vi "PH_PILS.set HV Warnlamp.vi"(0 "i ref in":refnum<vi>, 5 "error in (no error)":errorcluster) -> (14 "i ref out":refnum<vi>, 19 "error out":errorcluster)   [LabVIEW 2014, in "PH_PILS.lvlib"]
doc: "This VI switches flash lamp above door of the the HV-room in case of that the evacuation acqunoledgement is switched."
uses:
  PH_PILS.lvlib
  PH_Devices/PH_Beckhoff_PPMA-Rods/PH_Beckhoff_PPMA-Rods.lvlib
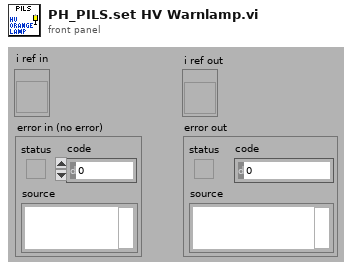
[diagram p1: front panel]
types:
  T1 = typedef "PH_PILS.lvlib/PH_PILS.i attribute.ctl" = cluster{"Boolean":cluster{"GUI Ref":refnum<vi>, "Status":i32}[], "GUI Refs Exp. Shutters":cluster{"1":refnum<vi>, "2":refnum<vi>, "3":refnum<vi>, "4":refnum<vi>}, "Tristate2Run GUI Refs":refnum<vi>[], "EO-Likes":cluster{"GUI Ref":refnum<vi>, "Status":i32}[], "Operation Mode":cluster{"Operation Mode":T2, "GUI":cluster{"Ref State":refnum<vi>, "Ref":refnum<vi>}, "Servicemode":cluster{"Tagname":string, "Status":i32}, "Labormode":cluster{"Tagname":string, "Status":i32}, "Searchmode":cluster{"Tagname":string, "Status":i32}, "Shotmode":cluster{"Tagname":string, "Status":i32}}, "Submode":cluster{"Submode":T3, "GUI":cluster{"Ref State":refnum<vi>, "Ref":refnum<vi>}, "Submode":cluster{"Tagname":string, "Status":i32}}, "Experiment":cluster{"Experiment":enum16{"unknown", "intern", "4 (Z6)", "3", "2", "1"}, "GUI":cluster{"Ref State":refnum<vi>, "Ref":refnum<vi>}, "intern":cluster{"Tagname":string, "Status":i32}, "Exp 4":cluster{"Tagname":string, "Status":i32}, "Exp 3":cluster{"Tagname":string, "Status":i32}, "Exp 2":cluster{"Tagname":string, "Status":i32}, "Exp 1":cluster{"Tagname":string, "Status":i32}}, "TristateNormal":cluster{"GUI Ref":refnum<vi>, "Status":i32}[], "Door Tags":cluster{"GUI Ref":refnum<vi>, "Status":i32}[], "GUIlessTags":cluster{"Name":string, "Status":i32}[], "Beamline GUI Refs":refnum<vi>[], "Special Boolean":cluster{"GUI Ref":refnum<vi>, "Status":i32}[], "Laserpower":cluster{"GUI Ref":refnum<vi>, "Status":i32}[], "Shutter":cluster{"GUI Ref":refnum<vi>, "Status":i32}[], "Tristate EO Like":cluster{"GUI Ref":refnum<vi>, "Status":i32}[], "PP":cluster{"GUI Ref":refnum<vi>, "Status":i32, "Head Ref":refnum<vi>, "Slider Ref":refnum<vi>}[], "Switch Knobs":cluster{"GUI Ref":refnum<vi>, "Status":i32}[], "Latch Knob GUI Refs":refnum<vi>[], "FailureCounter":i32, "Enabled Status":cluster{"Laser":i32, "PreAmp":i32, "MainAmp":i32}, "Mercury":refnum<vi>, "Instance Rods":string, "Logfile":path, "Beckhoff-Instance Internal":string, "Beckhoff-Instance External":string, "Enabling Rights":cluster{"Name":string, "Password":string, "PA?":bool, "MA?":bool, "Exp?":bool}[]}
  T2 = typedef "PH_PILS.lvlib/PH_PILS.Operation Mode.ctl" = enum16{"unknown", "Service", "Labor", "Search", "Shot"}
  T3 = typedef "PH_PILS.lvlib/PH_PILS.Submode.ctl" = enum16{"unknown", "HV-Normal", "HV-Test"}
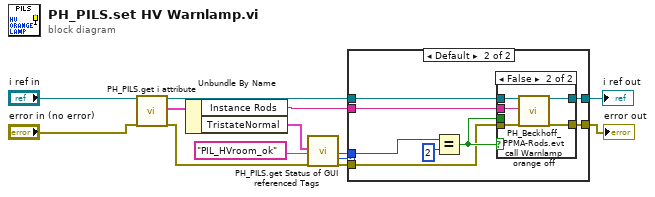
[diagram p0: block diagram]
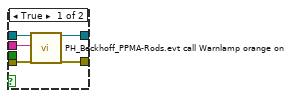
[diagram p3: hidden frame]
diagram:
  n1 = call "PH_PILS.get i attribute.vi"("i ref in"="i ref in", "error in (no error)"="error in (no error)") -> ("i ref out"=w3:refnum<vi>, "i attribute"=w13:T1, "error out"=w2:errorcluster)  [unwired: 15 in]
  n2 = Unbundle By Name(w13) -> ("Instance Rods"=w1:string, "TristateNormal"=w8:cluster{"GUI Ref":refnum<vi>, "Status":i32}[])
  n3 = call "PH_PILS.get Status of GUI referenced Tags.vi"("Tags"=w8, "Tagname"="PIL_HVroom_ok" ("DSC Int Proc"), "error in"=w2) -> ("Status"=w4:i32, "index of element"=w6:i32, "error out"=w5:errorcluster)  [unwired: 13 in, 1 out]
  n4 = case shown="Default" w6 {
    tunnel: w3 -> [w15 w22]
    tunnel: [w15 w21] -> w9
    tunnel: [w14 w20] -> w10
    tunnel: w5 -> [w14 w17]
    tunnel: w4 -> [_ w19]
    tunnel: w1 -> [_ w16]
    frame -1 {
    }
    frame Default {
      n5 = Equal?(x=w19, y=2) -> (x = y?=w18:bool)
      n6 = case shown="False" w18 {
        tunnel: w22 -> [w28 w33]
        tunnel: [w27 w32] -> w21
        tunnel: [w26 w31] -> w20
        tunnel: w17 -> [w25 w30]
        tunnel: w16 -> [w24 w29]
        tunnel: w18 -> [_ _]
        frame True {
          n7 = call "PH_Beckhoff_PPMA-Rods.evt call Warnlamp orange on.vi"("i ref in"=w28, "Instance name"=w24, "error in"=w25) -> ("i ref out"=w27:refnum<vi>, "error out"=w26:errorcluster)  [unwired: 15 in]
        }
        frame False {
          n8 = call "PH_Beckhoff_PPMA-Rods.evt call Warnlamp orange off.vi"("i ref in"=w33, "Instance name"=w29, "error in"=w30) -> ("i ref out"=w32:refnum<vi>, "error out"=w31:errorcluster)  [unwired: 15 in]
        }
      }
    }
  }
  "i ref out" <- w9
  "error out" <- w10
